vi "CreateHTML.vi"(0 "reference in":refnum<class "BooleanControl.lvclass">, 2 "VI Name":string, 5 "error in (no error)":errorcluster) -> (13 "script dependencies":string[](array[string]), 14 "reference out":refnum<class "BooleanControl.lvclass">, 15 "HTML":string, 16 "js variables":string, 17 "js code for controls":string, 18 "js code for indicators":string, 19 "error out":errorcluster)   [LabVIEW 2014, in "FrontPanelPublisher.lvlib" / "BooleanControl.lvclass"]
uses:
  BooleanControl.lvclass
  Text_class/Text.lvclass
  Object_class/Object.lvclass
  Control_class/Control.lvclass
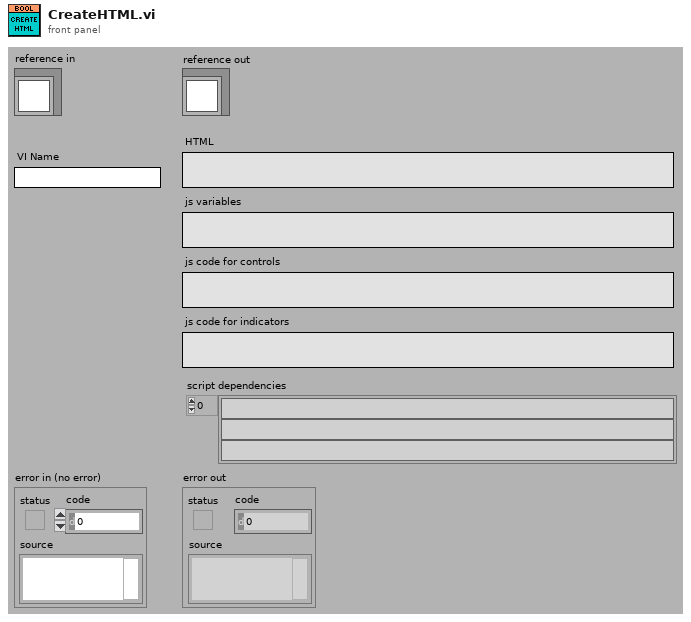
[diagram p1: front panel]
types:
  T1 = typedef "FrontPanelPublisher.lvlib/Object.lvclass/Attributes.ctl" = cluster{"UID":i32, "Type":string, "Coordinates":T2, "Reference":refnum<vi>}
  T2 = typedef "FrontPanelPublisher.lvlib/Object.lvclass/Coordinates.ctl" = cluster{"Left":i32, "Top":i32, "Height":u32, "Width":u32}
  T3 = typedef "FrontPanelPublisher.lvlib/Control.lvclass/Attributes.ctl" = cluster{"Description":string, "Indicator":bool, "Default Value":variant, "Control Index":i32, "Label":refnum<class "Text.lvclass">, "Caption":refnum<class "Text.lvclass">, "Use Picture":bool, "Image1 b64":string, "Image2 b64":string}
  T4 = typedef "FrontPanelPublisher.lvlib/BooleanControl.lvclass/Attributes.ctl" = cluster{"Boolean ref":refnum<vi>, "Switching":bool, "Boolean Strings":string[], "Text":refnum<class "Text.lvclass">}
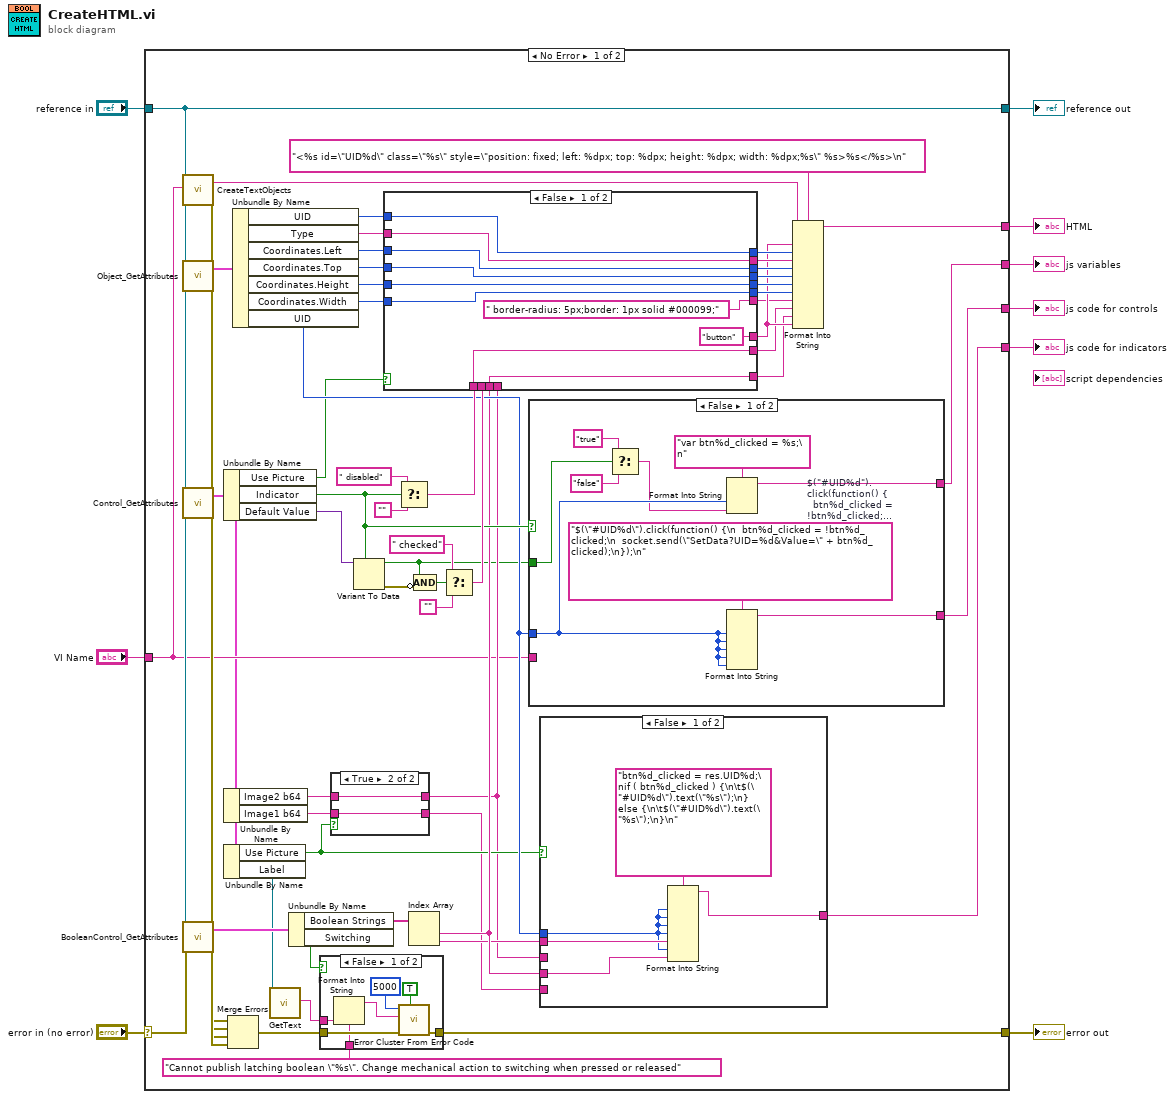
[diagram p0: block diagram]
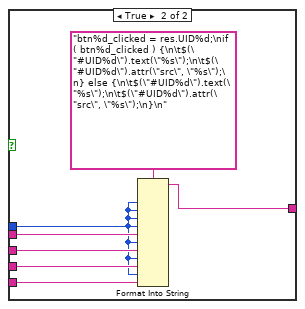
[diagram p4: hidden frame]
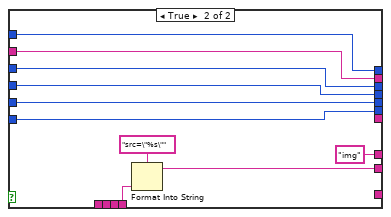
[diagram p6: hidden frame]
diagram:
  n1 = case shown="No Error" "error in (no error)" {
    selector: "error in (no error)" -> [w68 w121]
    tunnel: [w10 w121] -> w8
    tunnel: [w16 w120] -> w6
    tunnel: "reference in" -> [w16 w120]
    tunnel: [w60 _] -> w5
    tunnel: [w35 _] -> w4
    tunnel: [w34 _] -> w3
    tunnel: [w30 _] -> w2
    tunnel: "VI Name" -> [w15 _]
    frame No Error {
      n2 = call-dynamic "CreateTextObjects.vi"("reference in"=w16, "VI Name"=w15) -> ("HTML"=w14:string, "error out"=w62:errorcluster)  [unwired: 15 in, 1 out]
      n3 = call "Object_GetAttributes.vi"("reference in"=w16) -> ("Data"=w59:T1, "error out"=w63:errorcluster)  [unwired: 15 in, 2 out]
      n4 = call "Control_GetAttributes.vi"("reference in"=w16) -> ("Data"=w13:T3, "error out"=w64:errorcluster)  [unwired: 15 in, 2 out]
      n5 = call "BooleanControl_GetAttributes.vi"("reference in"=w16, "error in (no error)"=w68) -> ("Data"=w46:T4, "error out"=w66:errorcluster)  [unwired: 14 in, 2 out]
      n6 = Unbundle By Name(w13) -> ("Use Picture"=w27:bool, "Indicator"=w36:bool, "Default Value"=w39:variant)
      n7 = Unbundle By Name(w13) -> ("Image2 b64"=w12:string, "Image1 b64"=w11:string)
      n8 = Unbundle By Name(w13) -> ("Use Picture"=w24:bool, "Label"=w20:refnum<class "Text.lvclass">)
      n9 = Merge Errors(w62, w63, w64, w66) -> (w65:errorcluster)
      n10 = Unbundle By Name(w59) -> ("UID"=w58:i32, "Type"=w57:string, "Coordinates.Left"=w56:i32, "Coordinates.Top"=w55:i32, "Coordinates.Height"=w54:u32, "Coordinates.Width"=w53:u32, "UID"=w31:i32)
      n11 = call-dynamic "GetText.vi"("reference in"=w20) -> ("Text"=w19:string)  [unwired: 16 in, 2 out]
      n12 = Unbundle By Name(w46) -> ("Boolean Strings"=w37:string[], "Switching"=w17:bool)
      n13 = case shown="False" w17 {
        tunnel: [w75 w76] -> w10
        tunnel: w65 -> [w74 w76]
        tunnel: w19 -> [w71 _]
        tunnel: "Cannot publish latching boolean \"%s\". Change mechanical action to switching when pressed or released" -> [w70 _]
        frame False {
          n14 = Format Into String(format string=w70, w71) -> (resulting string=w69:string)  [unwired: 2 in, 1 out]
          n15 = call <vilib>:"Error Cluster From Error Code.vi"("show call chain? (False)"=TRUE, "error in (no error)"=w74, "error message (\"\")"=w69, "error code (0)"=5000) -> ("error out"=w75:errorcluster)  [unwired: 5 in]
        }
        frame True {
        }
      }
      n16 = case shown="True" w24 {
        tunnel: [_ w78] -> w22
        tunnel: [_ w77] -> w23
        tunnel: w12 -> [_ w78]
        tunnel: w11 -> [_ w77]
        frame False {
        }
        frame True {
        }
      }
      n17 = Variant To Data(type=w36, Variant=w39) -> (data=w21:bool, error out=w67:errorcluster)  [unwired: 1 in]
      n18 = Select(t=" disabled", s=w36, f="") -> (s? t:f=w43:string)
      n19 = Index Array(array=w37) -> (element #1=w29:string, element #2=w28:string)  [unwired: 2 in]
      n20 = Compound Arithmetic op=AND(w21, invert w67) -> (w42:bool)
      n21 = Select(t=" checked", s=w42, f="") -> (s? t:f=w38:string)
      n22 = case shown="False" w27 {
        tunnel: ["button" "img"] -> w33
        tunnel: w43 -> [w100 _]
        tunnel: w38 -> [_ _]
        tunnel: [w108 _] -> w32
        tunnel: w29 -> [w108 _]
        tunnel: [w100 w110] -> w25
        tunnel: [w106 w118] -> w51
        tunnel: w57 -> [w106 w118]
        tunnel: [w107 w117] -> w52
        tunnel: w58 -> [w107 w117]
        tunnel: [w105 w116] -> w50
        tunnel: w56 -> [w105 w116]
        tunnel: [w104 w115] -> w49
        tunnel: w55 -> [w104 w115]
        tunnel: [w102 w114] -> w47
        tunnel: w53 -> [w102 w114]
        tunnel: w54 -> [w103 w113]
        tunnel: [w103 w113] -> w48
        tunnel: [" border-radius: 5px;border: 1px solid #000099;" _] -> w26
        tunnel: w22 -> [_ w111]
        frame False {
        }
        frame True {
          n23 = Format Into String(format string="src=\"%s\"", w111) -> (resulting string=w110:string)  [unwired: 2 in, 1 out]
        }
      }
      n24 = case shown="False" w36 {
        tunnel: [w99 _] -> w34
        tunnel: w31 -> [w98 _]
        tunnel: [w97 _] -> w35
        tunnel: w15 -> [_ _]
        tunnel: w21 -> [w94 _]
        frame False {
          w96 = "$(\"#UID%d\").click(function() {\n  btn%d_clicked = !btn%d_clicked;\n  socket.send(\"SetData?UID=%d&Value=\" + btn%d_clicked);\n});\n"  # $("#UID%d").click(function() {   btn%d_clicked = !btn%d_clicked;   socket.send("SetData?UID=%d&Value=" + btn%d_clicked); });
          n25 = Select(t="true", s=w94, f="false") -> (s? t:f=w91:string)
          n26 = Format Into String(format string="var btn%d_clicked = %s;\n", w98, w91) -> (resulting string=w97:string)  [unwired: 2 in, 1 out]
          n27 = Format Into String(format string=w96, w98, w98, w98, w98, w98) -> (resulting string=w99:string)  [unwired: 2 in, 1 out]
        }
        frame True {
        }
      }
      n28 = case shown="False" w24 {
        tunnel: w28 -> [w83 w90]
        tunnel: w31 -> [w79 w84]
        tunnel: [w82 w89] -> w30
        tunnel: w29 -> [w80 w87]
        tunnel: w22 -> [_ w86]
        tunnel: w23 -> [_ w85]
        frame False {
          n29 = Format Into String(format string="btn%d_clicked = res.UID%d;\nif ( btn%d_clicked ) {\n\t$(\"#UID%d\").text(\"%s\");\n} else {\n\t$(\"#UID%d\").text(\"%s\");\n}\n", w79, w79, w79, w79, w83, w79, w80) -> (resulting string=w82:string)  [unwired: 2 in, 1 out]
        }
        frame True {
          n30 = Format Into String(format string="btn%d_clicked = res.UID%d;\nif ( btn%d_clicked ) {\n\t$(\"#UID%d\").text(\"%s\");\n\t$(\"#UID%d\").attr(\"src\", \"%s\");\n} else {\n\t$(\"#UID%d\").text(\"%s\");\n\t$(\"#UID%d\").attr(\"src\", \"%s\");\n}\n", w84, w84, w84, w84, w90, w84, w86, w84, w87, w84, w85) -> (resulting string=w89:string)  [unwired: 2 in, 1 out]
        }
      }
      n31 = Format Into String(format string="<%s id=\"UID%d\" class=\"%s\" style=\"position: fixed; left: %dpx; top: %dpx; height: %dpx; width: %dpx;%s\" %s>%s</%s>\n", initial string=w14, w33, w52, w51, w50, w49, w48, w47, w26, w25, w32, w33) -> (resulting string=w60:string)  [unwired: 1 in, 1 out]
    }
    frame Error {
    }
  }
  "error out" <- w8
  "reference out" <- w6
  "HTML" <- w5
  "js variables" <- w4
  "js code for controls" <- w3
  "js code for indicators" <- w2
